vi "NT Server mod.vi"(6 "Update Time":i32=100, 8 "error in (no error)":errorcluster, 9 "Timeout":i32=1000, 10 "Server Name":string, 11 "Enable Read Errors":bool) -> ()   [LabVIEW 2014]
doc: "Place this VI into the robot code so that it can run in parallel with the rest of the code. The top level of Robot Main is a good location. You may then read and write as many variables to as many tables as you need."
uses:
  <vilib>/Rock Robotics/WPI/DriverStation/WPI_DriverStationRobotMode2.ctl
  <vilib>/Rock Robotics/Network Tables/NT Globals.vi
panel:
  in  "stop":bool
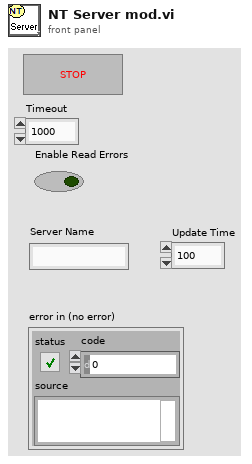
[diagram p1: front panel]
types:
  T1 = typedef "WPI_DriverStationRobotMode2.ctl" = enum16{"Autonomous Disabled", "Autonomous Enabled", "Teleop Disabled", "Teleop Enabled", "Disconnected", "Finish", "Test Disabled", "Test Enabled", "Emergency Stopped"}
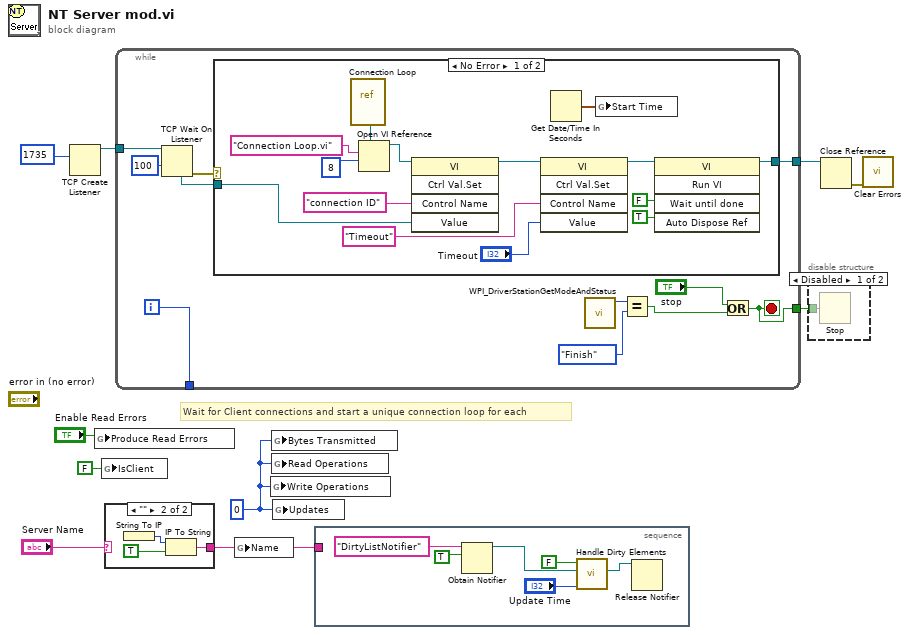
[diagram p0: block diagram]
diagram:
  w5 = 0 ("Updates")
  # "Wait for Client connections and start a unique connection loop for each"
  n1 = TCP Create Listener(10:u16 1735 ("port")) -> (3:w9:refnum<k5>)  [unwired: 4 in, 2 out]
  n2 = global write "NT Globals.vi" "Produce Read Errors"("Enable Read Errors") -> ()
  n3 = global write "NT Globals.vi" "IsClient"(FALSE ("IsClient")) -> ()
  n4 = case shown="\"\"" "Server Name" {
    selector: "Server Name" -> [w11 _]
    tunnel: [w11 w12] -> w3
    frame Default {
    }
    frame "" {
      n5 = String To IP() -> (0:w14:u32)  [unwired: 1 in]
      n6 = IP To String(1:TRUE ("dot notation? (F)"), 2:w14) -> (0:w12:string)
    }
  }
  n7 = while {
    tunnel: w9 -> [w25]
    tunnel: [w23] -> _
    tunnel: [w22] -> w7
    tunnel: [w15] -> w1
    i -> [w23]
    stop <- w15 stop-if-true
    n8 = TCP Wait On Listener(9:100 ("timeout ms (wait forever: -1)"), 11:w25) -> (0:w21:errorcluster, 4:w24:refnum<k5>)  [unwired: 2 in, 3 out]
    n9 = case shown="No Error" w21 {
      tunnel: w24 -> [w38 _]
      tunnel: [w34 _] -> w22
      frame No Error {
        n10 = vi-ref <vilib>:"Connection Loop.vi"() -> (w30:refnum<vi>)
        n11 = Open VI Reference(type specifier VI Refnum (for type only)=w30, vi path="Connection Loop.vi", options=8) -> (vi reference=w32:refnum<vi>)  [unwired: 3 in, 1 out]
        n12 = invoke class="VI" method="Ctrl Val.Set"(reference=w32, "Control Name"="connection ID", "Value"=w38) -> (reference out=w29:refnum<vi>)  [unwired: 2 in, 4 out]
        n13 = invoke class="VI" method="Ctrl Val.Set"(reference=w29, "Control Name"="Timeout", "Value"="Timeout") -> (reference out=w28:refnum<vi>)  [unwired: 2 in, 4 out]
        n14 = Get Date/Time In Seconds() -> (seconds since 1Jan1904=w39:timestamp)
        n15 = global write "NT Globals.vi" "Start Time"(w39) -> ()
        n16 = invoke class="VI" method="Run VI"(reference=w28, "Wait until done"=FALSE ("Wait Until Done"), "Auto Dispose Ref"=TRUE ("Auto Dispose Reference")) -> (reference out=w34:refnum<vi>)  [unwired: 2 in, 4 out]
      }
      frame Error {
      }
    }
    n17 = call <vilib>:"WPI_DriverStationGetModeAndStatus.vi"() -> ("Robot Mode"=w19:T1)  [unwired: 10 in, 1 out]
    n18 = Equal?(x=w19, y=WPI_DriverStationRobotMode2."Finish") -> (x = y?=w16:bool)
    n19 = Or(x="stop", y=w16) -> (x .or. y?=w15:bool)
  }
  n20 = global write "NT Globals.vi" "Name"(w3) -> ()
  n21 = global write "NT Globals.vi" "Write Operations"(w5) -> ()
  n22 = global write "NT Globals.vi" "Bytes Transmitted"(w5) -> ()
  n23 = global write "NT Globals.vi" "Read Operations"(w5) -> ()
  n24 = global write "NT Globals.vi" "Updates"(w5) -> ()
  n25 = stacked-sequence {
    tunnel: w3 -> [_]
    frame #0 {
      n26 = Obtain Notifier(name (unnamed)="DirtyListNotifier", notification data type=TRUE ("IsClient")) -> (notifier out=w41:refnum<notifier>)  [unwired: 2 in, 2 out]
      n27 = call <vilib>:"Handle Dirty Elements.vi"("Update Time"="Update Time", "notifier out"=w41, "IsClient"=FALSE) -> ("notifier out 2"=w40:refnum<notifier>)  [unwired: 8 in]
      n28 = Release Notifier(notifier=w40) -> ()  [unwired: 2 in, 3 out]
    }
  }
  n29 = disable-structure shown="Disabled" {
    disable-tunnel: w1 -> [w46 _]
    frame Disabled {
      n30 = Stop(stop? (T)=w46) -> ()
    }
    frame Enabled {
    }
  }
  n31 = Close Reference(reference=w7) -> (error out=w2:errorcluster)  [unwired: 1 in]
  n32 = call <vilib>:"Clear Errors.vi"("error in (no error)"=w2) -> ()  [unwired: 5 in, 2 out]
